vi "initializeSR430.vi"(8 "error in (no error)":errorcluster, 10 "SR430 VISA Cluster":T1, 11 "dataClass in":refnum<class "SR430Class.lvclass">) -> (0 "error out":errorcluster, 1 "ID #:":string, 2 "Connected":bool, 3 "dataClass out":refnum<class "SR430Class.lvclass">)   [LabVIEW 2015, in "SR430Class.lvclass"]
uses:
  class/SR430Class.lvclass
  support/SR430 Driver/SR430_VISA Control.ctl
  class/SR430Class.lvclass/SR430Class.ctl
  support/SR430 Driver/SR430Driver.lvlib
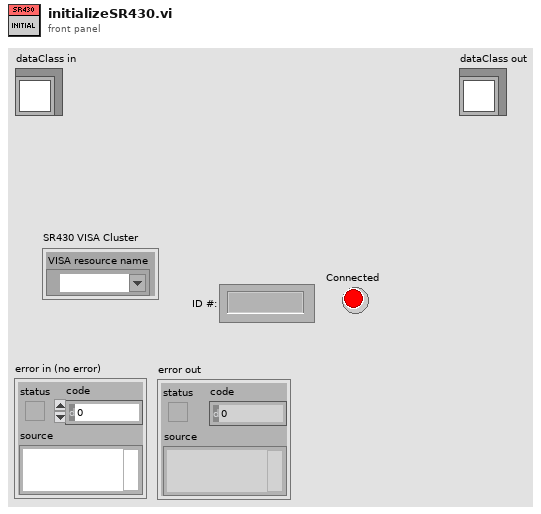
[diagram p1: front panel]
types:
  T1 = typedef "SR430Driver.lvlib/SR430_VISA Control.ctl" = cluster{"VISA resource name":refnum<visa-resource-name>}
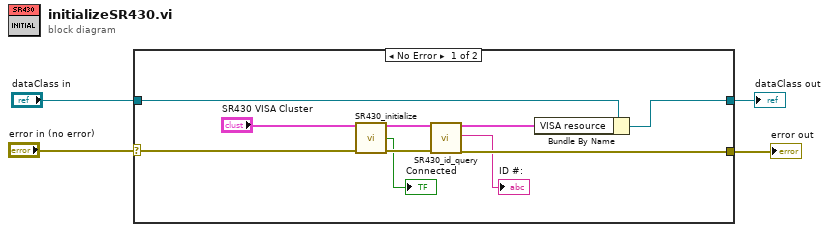
[diagram p0: block diagram]
diagram:
  n1 = case shown="No Error" "error in (no error)" {
    selector: "error in (no error)" -> [w12 w16]
    tunnel: [w11 w16] -> w3
    tunnel: [w7 w15] -> w1
    tunnel: "dataClass in" -> [w8 w15]
    frame No Error {
      n2 = call "SR430_initialize.vi"("SR430 VISA Cluster"="SR430 VISA Cluster", "error in (no error)"=w12) -> ("SR430 VISA Cluster out"=w14:T1, "interface initialized"=→"Connected":bool, "error out"=w13:errorcluster)  [unwired: 10 in, 1 out]
      n3 = call "SR430_id_query.vi"("address"=w14, "error in (no error)"=w13) -> ("address out"=w6:T1, "identification string"=→"ID #:":string, "error out"=w11:errorcluster)  [unwired: 15 in]
      n4 = Bundle By Name(cluster=w8, "VISA resource"=w6) -> (w7:refnum<class "SR430Class.lvclass">)
    }
    frame Error {
    }
  }
  "error out" <- w3
  "dataClass out" <- w1
